vi "ParseKeys.vi"(7 "desired":string[](array[string]), 8 "error in (no error)":errorcluster, 11 "reply":string) -> (0 "error out":errorcluster, 2 "menu":string[](array[string]), 3 "Chart":i32(graph), 5 "Chart 2":i32[][](graph))   [LabVIEW 2024]
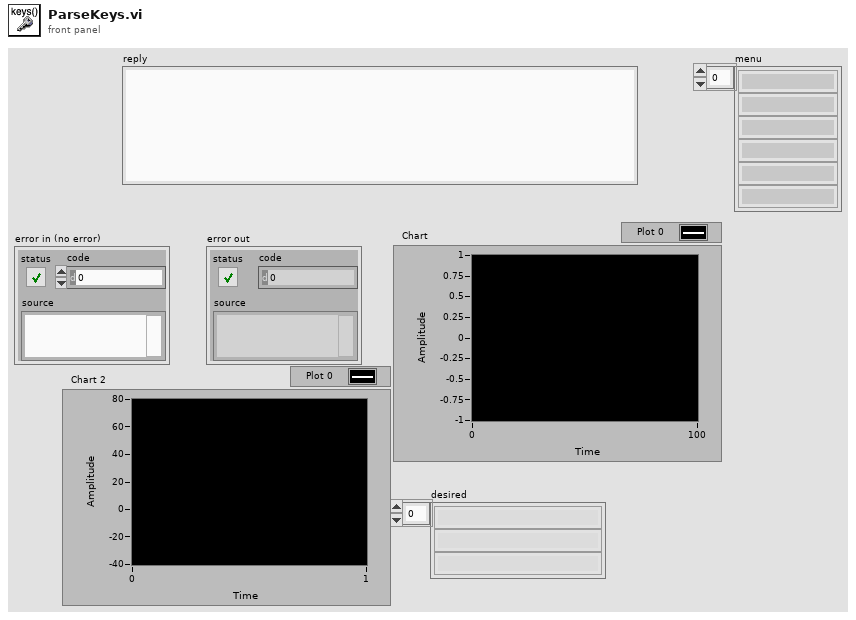
[diagram p1: front panel]
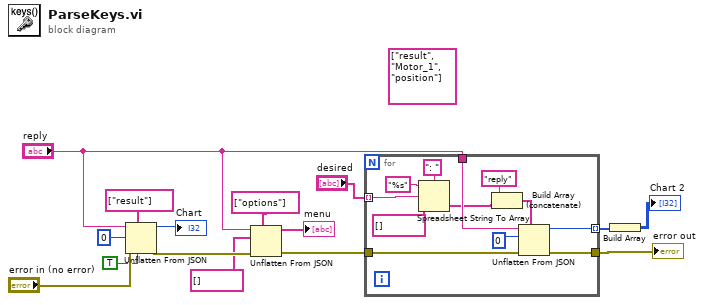
[diagram p0: block diagram]
diagram:
  (unwired) string[] ["result", "Motor_1", "position"] ("path")
  n1 = Unflatten From JSON(path=string[] ["result"], JSON string="reply", type and defaults=0 ("milliseconds to wait"), default null elements? (F)=TRUE, error in (no error)="error in (no error)") -> (value=→"Chart":i32, error out=w12:errorcluster)  [unwired: 2 in]
  n2 = Unflatten From JSON(path=string[] ["options"], JSON string="reply", type and defaults=string[] [], error in (no error)=w12) -> (value=→"menu":string[], error out=w3:errorcluster)  [unwired: 3 in]
  n3 = for {
    tunnel: "desired" -> [w27] mode=indexing
    tunnel: "reply" -> [w23]
    tunnel: [w21] -> w5 mode=indexing
    tunnel: w3 -> [w17]
    tunnel: [w16] -> w2
    n4 = Spreadsheet String To Array(delimiter (Tab)=": ", format string="%s", spreadsheet string=w27, array type (2D Dbl)=string[] []) -> (array=w19:string[])
    n5 = Build Array (concatenate)("reply", w19) -> (w18:string[])
    n6 = Unflatten From JSON(path=w18, JSON string=w23, type and defaults=0 ("milliseconds to wait"), error in (no error)=w17) -> (value=w21:i32, error out=w16:errorcluster)  [unwired: 3 in]
  }
  "error out" <- w2
  n7 = Build Array(w5) -> (→"Chart 2":i32[][])
